vi "Doc_Builder_Write_FrontPanel.vi"(10 "input item file path":path, 11 "NI_report in":refnum<class "NI_report.lvclass">) -> (3 "NI_report out":refnum<class "NI_report.lvclass">)   [LabVIEW 2019]
uses:
  <vilib>/Utility/NIReport.llb/NI_report.lvclass
  <vilib>/Utility/NIReport.llb/HTML Report Image Alignment.ctl
  <vilib>/printing/ReportDocExtensions.llb/Append Front Panel Image to Report (path).vi
  <vilib>/Utility/NIReport.llb/NI_ReportGenerationCore.lvlib
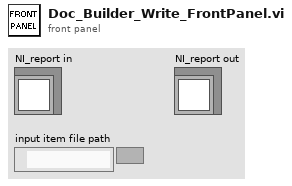
[diagram p1: front panel]
types:
  T1 = typedef "NI_ReportGenerationCore.lvlib/HTML Report Image Alignment.ctl" = enum16{"(default)", "LEFT", "RIGHT", "TOP", "TEXTTOP", "MIDDLE", "ABSMIDDLE", "BASELINE", "BOTTOM", "ABSBOTTOM"}
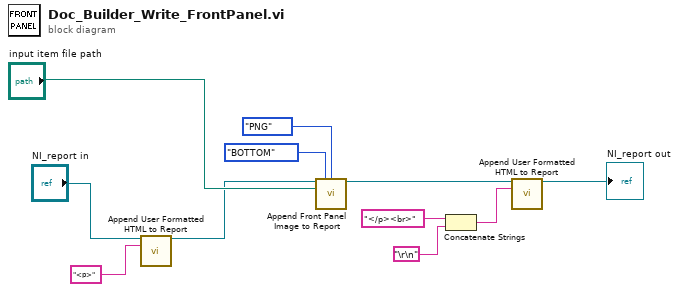
[diagram p0: block diagram]
diagram:
  n1 = call-dynamic "Append User Formatted HTML to Report.vi"("report in"="NI_report in", "HTML text"="<p>" ("text")) -> ("report out"=w1:refnum<class "NI_report.lvclass">)  [unwired: 12 in, 1 out]
  n2 = call-poly <vilib>:"Append Front Panel Image to Report.vi"("report in"=w1, "alignment (default)"=HTML_Report_Image_Alignment."BOTTOM", "image format (jpeg)"=enum32{"PNG", "JPEG", "GIF"}."PNG", "VI"="input item file path") -> ("report out"=w5:refnum<class "NI_report.lvclass">)  [unwired: 7 in, 4 out]
  n3 = Concatenate Strings("</p><br>" ("text"), "\r\n") -> (w6:string)
  n4 = call-dynamic "Append User Formatted HTML to Report.vi"("report in"=w5, "HTML text"=w6) -> ("report out"=→"NI_report out":refnum<class "NI_report.lvclass">)  [unwired: 12 in, 1 out]
